vi "AVS_SetOemParameter.vi"(2 "a_pOemData":u8[](array[numeric]), 3 "a_hDevice":i32) -> (0 "a_pOemData":u8[](array[numeric]), 1 "Output Value":i32)   [LabVIEW 2009]
uses:
  avaspecx64.dll
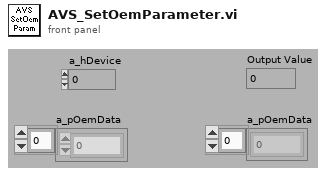
[diagram p1: front panel]
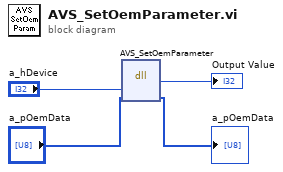
[diagram p0: block diagram]
diagram:
  n1 = dll-call lib="E:/libraries/Avaspec_Library/demo_64bit/LabView/LabViewSingleChan/avaspecx64.dll" fn="AVS_SetOemParameter" ("AS5216.dll:AVS_SetParameter")("a_hDevice"="a_hDevice", "a_pOemdata"="a_pOemData") -> ("return type"=→"Output Value":i32, "a_pOemdata"=→"a_pOemData":u8[])  [unwired: 4 in, 2 out]
